vi "Ej_7_Generador_Histograma.vi"() -> ()   [LabVIEW 2021]
uses:
  <vilib>/Instr/_visa.llb/VISA Configure Serial Port (Instr).vi
panel:
  out "Promedio":dbl
  out "Fuera de rango":bool
  out "min(x,y)":dbl
  out "max(x,y)":dbl
  out "number":dbl
  in  "stop":bool
  in  "VISA resource name":refnum<visa-resource-name>
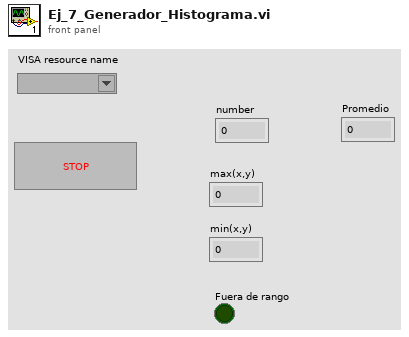
[diagram p1: front panel]
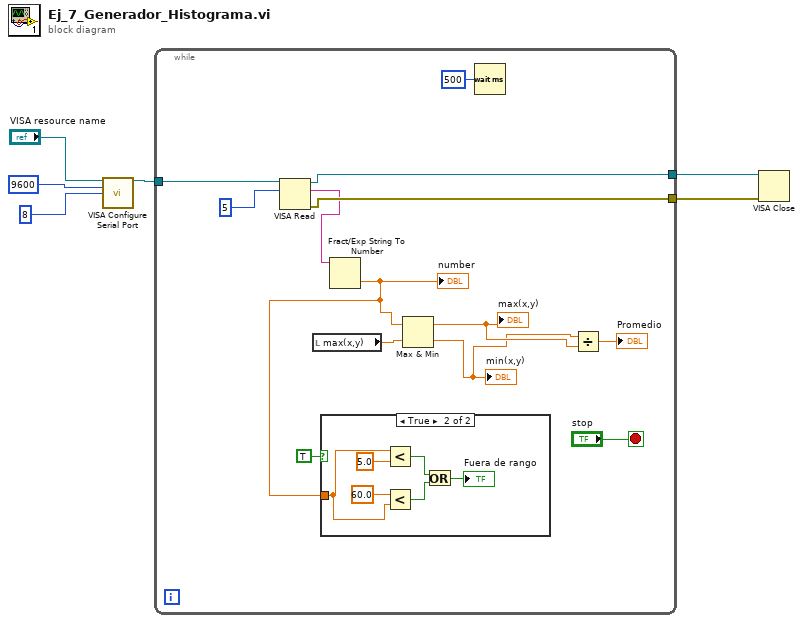
[diagram p0: block diagram]
diagram:
  n1 = call-poly "VISA Configure Serial Port"("VISA resource name"="VISA resource name", "baud rate (9600)"=u32 9600, "data bits (8)"=u16 8) -> ("VISA resource name out"=w3:refnum<visa-resource-name>)  [unwired: 11 in, 1 out]
  n2 = while {
    tunnel: w3 -> [w19]
    tunnel: [w15] -> w2
    tunnel: [w14] -> w1
    stop <- "stop" stop-if-true
    n3 = VISA Read(VISA resource name=w19, byte count=u32 5) -> (VISA resource name out=w15:refnum<visa-resource-name>, read buffer=w13:string, error out=w14:errorcluster)  [unwired: 1 in, 1 out]
    n4 = local read "max(x,y)"() -> (w12:dbl)
    n5 = Fract/Exp String To Number(string=w13) -> (number=w9:dbl)  [unwired: 3 in, 1 out]
    "number" <- w9
    n6 = case shown="True" TRUE {
      tunnel: w9 -> [_ w25]
      frame False {
      }
      frame True {
        n7 = Less?(x=w25, y=5.0) -> (x < y?=w21:bool)
        n8 = Less?(x=60.0, y=w25) -> (x < y?=w20:bool)
        n9 = Or(x=w21, y=w20) -> (x .or. y?=→"Fuera de rango":bool)
      }
    }
    n10 = Max & Min(x=w9, y=w12) -> (max(x,y)=w8:dbl, min(x,y)=w7:dbl)
    "max(x,y)" <- w8
    "min(x,y)" <- w7
    n11 = Wait (ms)(milliseconds to wait=u32 500) -> ()  [unwired: 1 out]
    n12 = Divide(x=w7, y=w8) -> (x/y=→"Promedio":dbl)
  }
  n13 = VISA Close(VISA resource name=w2, error in (no error)=w1) -> ()  [unwired: 1 out]
